vi "BME_DG_ReleaseMemory.vi"(8 "error in (no error)":errorcluster) -> (0 "error out":errorcluster, 3 "return code":i32)   [LabVIEW 2009, in "POLARIS BME DG.lvlib"]
uses:
  POLARIS BME DG.lvlib
  BME DLL/DelayGenerator.dll
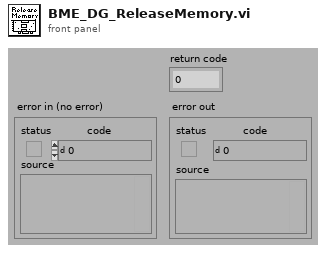
[diagram p1: front panel]
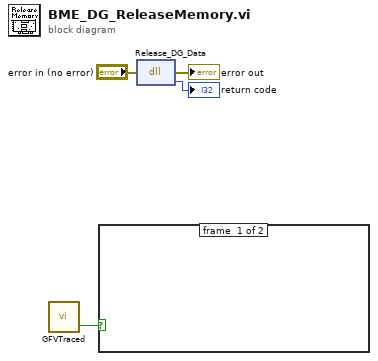
[diagram p0: block diagram]
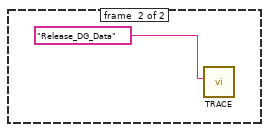
[diagram p2: hidden frame]
diagram:
  n1 = call "GFVTraced.vi"() -> ("traced?"=w1:bool)  [unwired: 2 in]
  n2 = case shown="True" w1 {
    frame #0 {
    }
    frame #1 {
      n3 = call "TRACE.vi"("Function"="Release_DG_Data") -> ()  [unwired: 11 in]
    }
  }
  n4 = dll-call lib="D:/CS Framework/LVSCC/LV2009/GPL/Projects/cs-framework/CSClass/CSPOLARIS/POLARIS BME DG/BME DLL/DelayGenerator.dll" fn="Release_DG_Data"(error in="error in (no error)") -> (error out=→"error out":errorcluster, →"return code":i32)  [unwired: 2 in, 1 out]
